vi "Save Button Info.vi"(10 "control info":T1[](array[typedef]) {"Boolean Type" items=["N/A", "FAB--icon--rounded", "outline--icon--rectangular", "outline--icon--rounded", "outline--text--rectangular", "outline--text--rounded", "nooutline--icon--rectangular", "nooutline--icon--rectangular--40x40", "nooutline--icon--rounded", "nooutline--text--rectangular", "nooutline--text--rounded", "tonal--icon--rectangular", "tonal--icon--rounded", "tonal--text--rectangular", "tonal--text--rounded", "filled--icon--rectangular", "filled--icon--rounded", "filled--text--rectangular", "filled--text--rounded"]; "UI Theme Level" items=["N/A", "Primary", "Secondary", "Tertiary", "Error", "Primary Fixed", "Secondary Fixed", "Tertiary Fixed", "Label Only", "No Change"]}, 11 "map in":map{string, refnum<vi>}(c390)) -> (0 "error out":errorcluster)   [LabVIEW 2021]
uses:
  control info.ctl
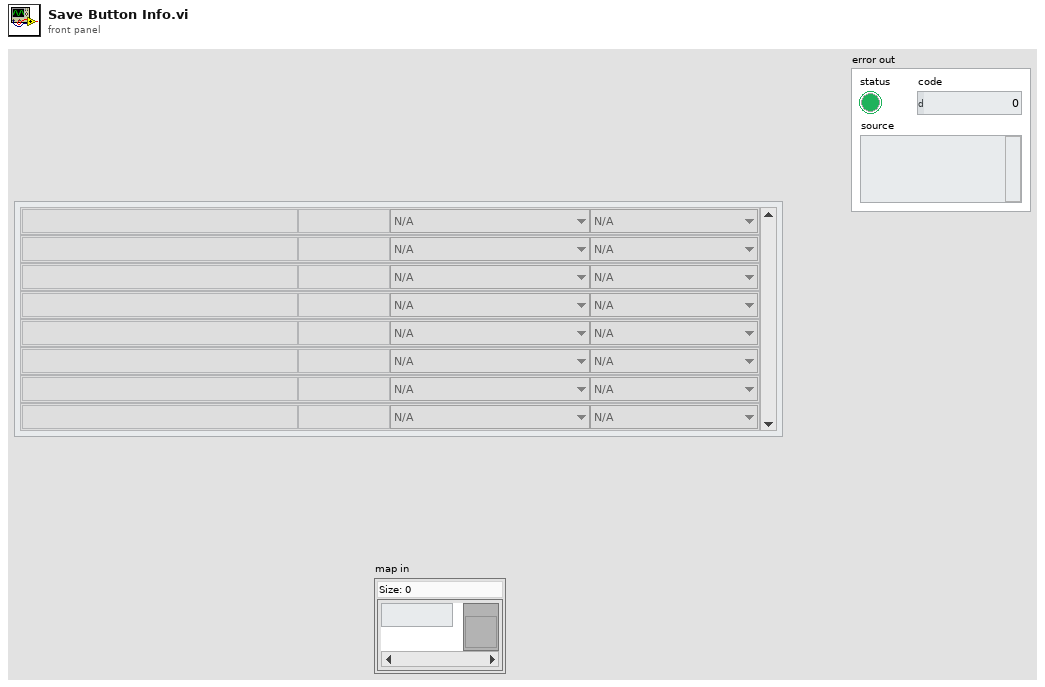
[diagram p1: front panel]
types:
  T1 = typedef "control info.ctl" = cluster{"label":string, "control type":string, "UI Theme Level":u16, "Boolean Type":u16}
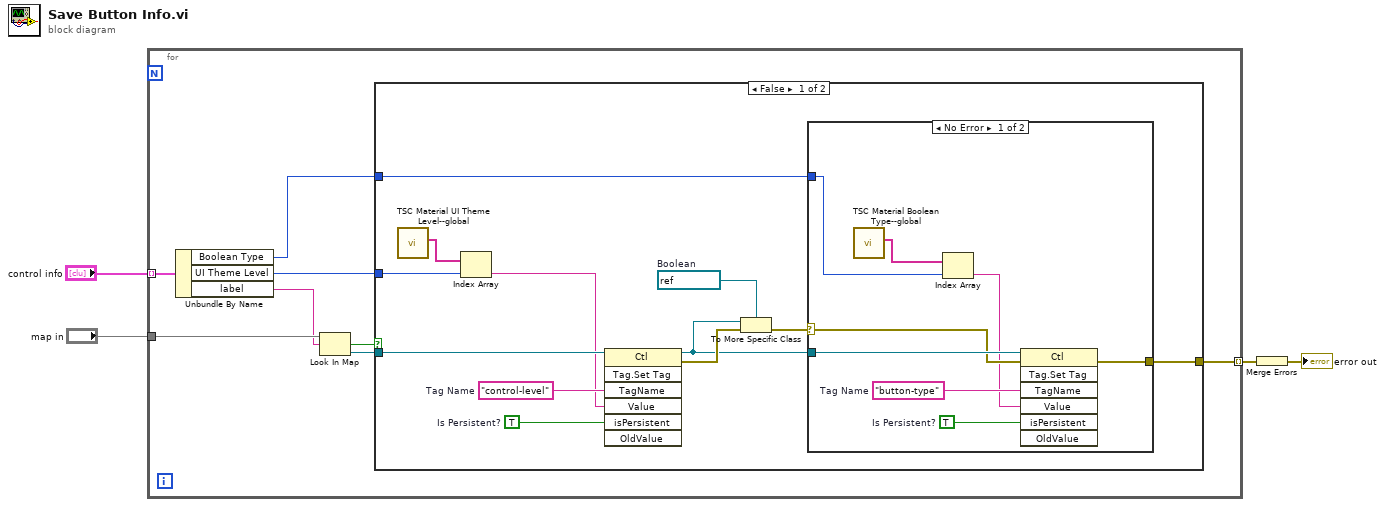
[diagram p0: block diagram]
diagram:
  n1 = for {
    tunnel: "map in" -> [w12]
    tunnel: "control info" -> [w11] mode=indexing
    tunnel: [w5] -> w2 mode=indexing
    n2 = Unbundle By Name(w11) -> ("Boolean Type"=w6:u16, "UI Theme Level"=w7:u16, "label"=w10:string)
    n3 = Look In Map(map=w12, key=w10) -> (key not found?=w9:bool, value=w8:refnum<vi>)  [unwired: 1 in]
    n4 = case shown="False" w9 {
      tunnel: w8 -> [w20 _]
      tunnel: w7 -> [w23 _]
      tunnel: w6 -> [w13 _]
      tunnel: [w14 _] -> w5
      frame False {
        w17 = refnum<vi> refnum  # Boolean
        w21 = TRUE  # Is Persistent?
        w22 = "control-level"  # Tag Name
        n5 = call "TSC Material UI Theme Level--global.vi"() -> ("UI theme levels"=w24:string[])  [unwired: 11 in]
        n6 = Index Array(array=w24, index=w23) -> (element=w19:string)
        n7 = invoke class="Ctl" method="Tag.Set Tag"(reference=w20, "TagName"=w22, "Value"=w19, "isPersistent"=w21) -> (reference out=w15:refnum<vi>, error out=w18:errorcluster)  [unwired: 3 in, 5 out]
        n8 = To More Specific Class(target class=w17, reference=w15, error in=w18) -> (error out=w16:errorcluster)  [unwired: 1 out]
        n9 = case shown="No Error" w16 {
          selector: w16 -> [w31 _]
          tunnel: w15 -> [w32 _]
          tunnel: [w30 _] -> w14
          tunnel: w13 -> [w26 _]
          frame No Error {
            w28 = TRUE  # Is Persistent?
            w29 = "button-type"  # Tag Name
            n10 = call "TSC Material Boolean Type--global.vi"() -> ("boolean types"=w27:string[])  [unwired: 11 in]
            n11 = Index Array(array=w27, index=w26) -> (element=w25:string)
            n12 = invoke class="Ctl" method="Tag.Set Tag"(reference=w32, error in=w31, "TagName"=w29, "Value"=w25, "isPersistent"=w28) -> (error out=w30:errorcluster)  [unwired: 2 in, 6 out]
          }
          frame Error {
          }
        }
      }
      frame True {
      }
    }
  }
  n13 = Merge Errors(w2) -> (→"error out":errorcluster)
